vi "FindNrSteps.vi"(1 "X calibration":cluster{dbl, dbl}[](graph), 2 "pixels":dbl) -> (0 "NrSteps":dbl)   [LabVIEW 2013]
uses:
  <vilib>/Analysis/NI_AALPro.lvlib
panel:
  out "transposed array":dbl[][](array[numeric]) format="%.2f"
  out "Array NO duplicates":i32[][](array[numeric])
  out "Sorted array":dbl[][](array[numeric]) format="%.2f"
  out "steps":dbl[](array[numeric])
  out "pix (x in interpolant)":dbl[](array[numeric])
  out "error out":errorcluster
  out "Interpolant":dbl[](array[numeric]) format="%0.2f"
  out "error 2":i32
  out "error":i32
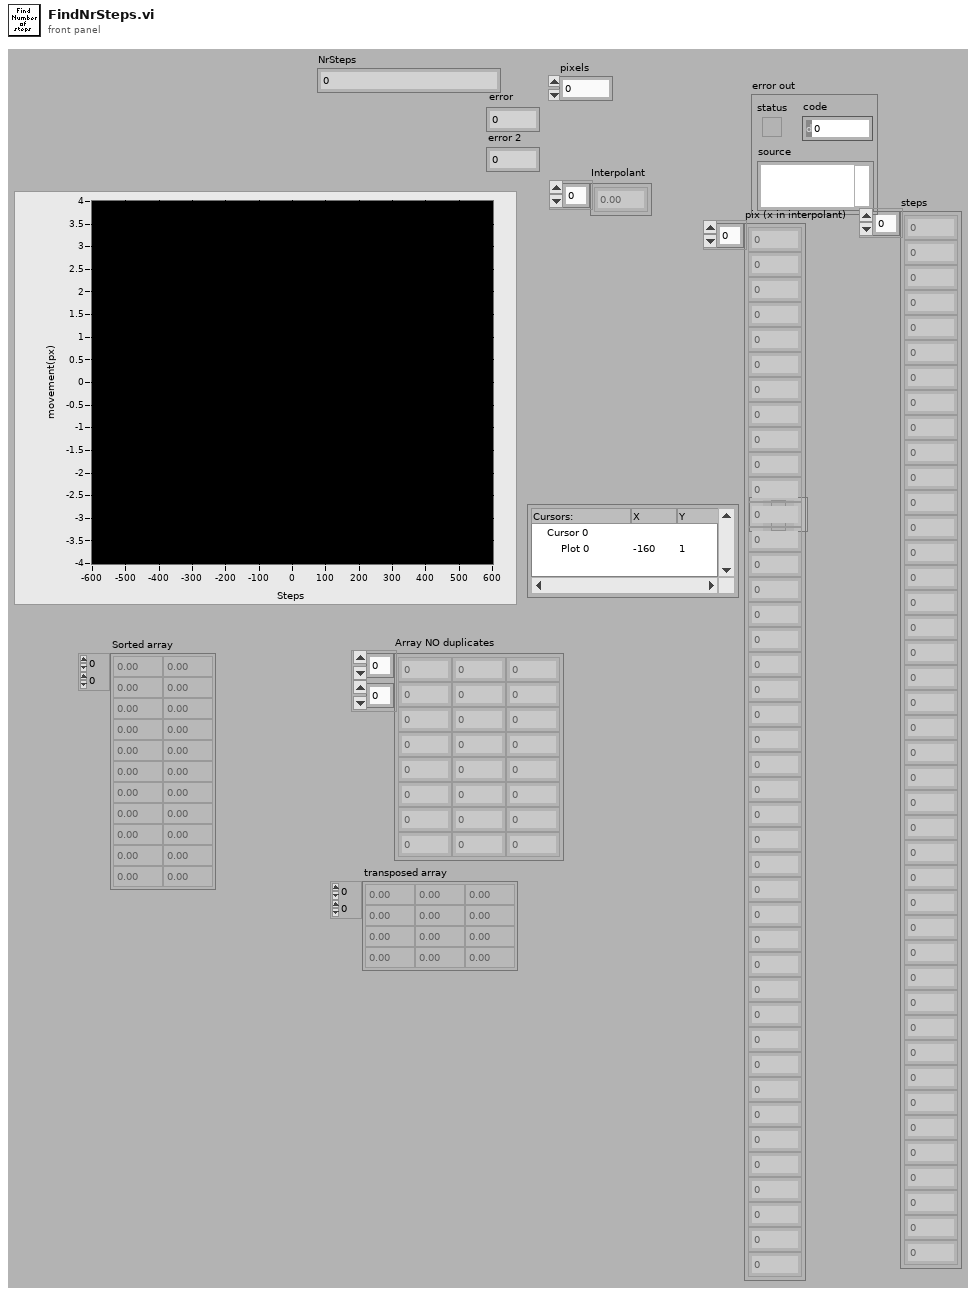
[diagram p1: front panel]
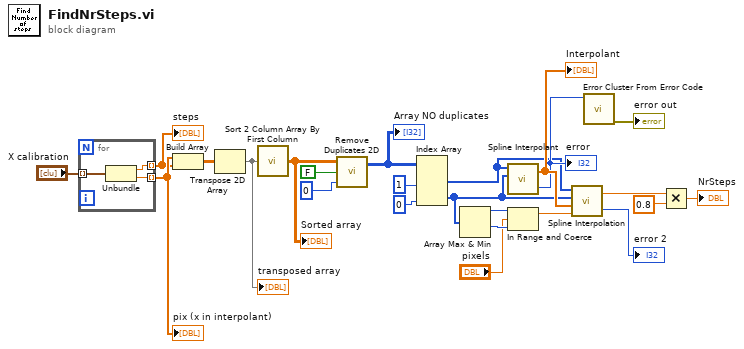
[diagram p0: block diagram]
diagram:
  n1 = for {
    tunnel: "X calibration" -> [w25] mode=indexing
    tunnel: [w27] -> w2 mode=indexing
    tunnel: [w26] -> w1 mode=indexing
    n2 = Unbundle(w25) -> (w26:dbl, w27:dbl)
  }
  "pix (x in interpolant)" <- w2
  "steps" <- w1
  n3 = Build Array(w2, w1) -> (w11:dbl[][])
  n4 = Transpose 2D Array(2D array=w11) -> (transposed array=w10:dbl[][])
  "transposed array" <- w10
  n5 = call "Sort 2 Column Array By First Column.vi"("2D array to sort"=w10) -> ("Sorted array"=w12:dbl[][])
  "Sorted array" <- w12
  n6 = call "Remove Duplicates 2D.vi"("Which column/row"=0, "By column/row"=FALSE, "Array in"=w12) -> ("Array out"=w7:i32[][])  [unwired: 1 out]
  "Array NO duplicates" <- w7
  n7 = Index Array(array=w7, index (col) #1=1 ("disabled index (col)"), index (col) #2=0 ("index (col)")) -> (element #1=w5:i32[], element #2=w4:i32[])  [unwired: 2 in]
  n8 = Array Max & Min(array=w4) -> (max value=w21:i32, min value=w20:i32)  [unwired: 2 out]
  n9 = call <vilib>:"Spline Interpolant.vi"("X"=w4, "Y"=w5) -> ("error"=w15:i32, "Interpolant"=w23:dbl[])  [unwired: 2 in]
  "error" <- w15
  "Interpolant" <- w23
  n10 = In Range and Coerce(upper limit=w21, x="pixels", lower limit=w20) -> (coerced(x)=w18:dbl)  [unwired: 1 out]
  n11 = call <vilib>:"Spline Interpolation.vi"("x value"=w18, "Interpolant"=w23, "X"=w4, "Y"=w5) -> ("error"=→"error 2":i32, "interpolation value"=w22:dbl)
  n12 = call <vilib>:"Error Cluster From Error Code.vi"("error code (0)"=w15) -> ("error out"=→"error out":errorcluster)  [unwired: 8 in]
  n13 = Multiply(x=w22, y=0.8) -> (x*y=→"NrSteps":dbl)
